vi "Sefram DAS220 - Configure and Read Channel.vi"() -> ()   [LabVIEW 2017, in "Sefram DAS220.lvlib"]
doc: "Configure an analog channel and read values."
uses:
  <instrlib>/Sefram DAS220/Sefram DAS220.lvlib
  <vilib>/Utility/error.llb/DialogType.ctl
  <instrlib>/Sefram DAS220/Public/Configure/Channels/Low-level/Set Type Voltage.vi
panel:
  in  "Channel":u16(ring) items=["A1"=0, "A2"=1, "A3"=2, "A4"=3, "A5"=4, "A6"=5, "A7"=6, "A8"=7, "A9"=8, "A10"=9, "K1"=200, "K2"=201, "K3"=202, "K4"=203, "FA1"=204, "FA2"=205, "FA3"=206, "FA4"=207]
  out "Channel":dbl(graph)
  in  "Center in Volt":dbl
  in  "Range in Volt":dbl=10.0 format="%#_13g"
  in  "stop":bool
  in  "VISA resource name":refnum<visa-resource-name>
  # "Channel Settings"
  # "Acquired Data"
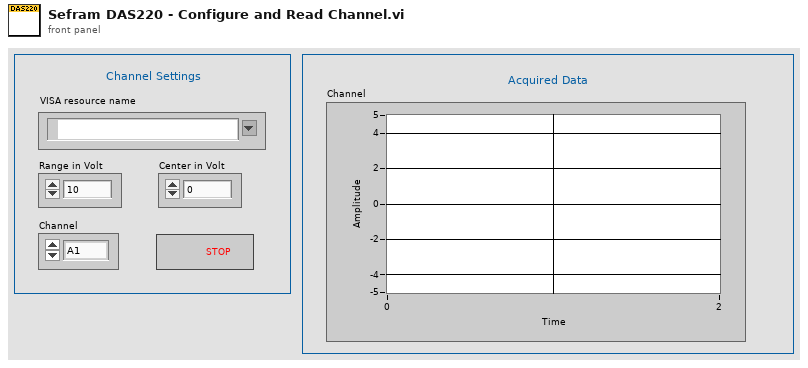
[diagram p1: front panel]
types:
  T1 = enum16{"open", "replace", "create", "open or create", "replace or create", "replace or create with confirmation"}
  T2 = typedef "DialogType.ctl" = u16
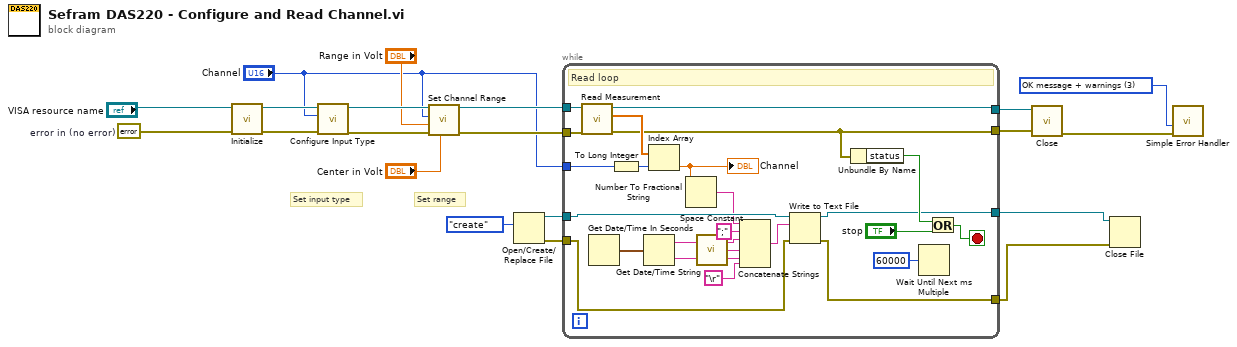
[diagram p0: block diagram]
diagram:
  w17 = errorcluster {"status"=FALSE, "code"=0, "source"=""}  # error in (no error)
  w15 = T2 3 items=["no dialog", "OK message", "continue or stop message", "OK message + warnings", "continue/stop + warnings"] ("type of dialog (OK msg:1)")
  # "Set range"
  # "Set input type"
  n1 = call <instrlib>:"Initialize.vi"("error in (no error)"=w17, "VISA resource name"="VISA resource name") -> ("error out"=w13:errorcluster, "VISA resource name out"=w14:refnum<visa-resource-name>)  [unwired: 8 in]
  n2 = call-poly <instrlib>:"Configure Input Type.vi"("error in (no error)"=w13, "Channel"="Channel", "VISA resource name"=w14) -> ("error out"=w11:errorcluster, "VISA resource name out"=w12:refnum<visa-resource-name>)  [unwired: 7 in]
  n3 = call <instrlib>:"Set Channel Range.vi"("Center (in actual channel unit)"="Center in Volt", "error in (no error)"=w11, "Channel range (in actual channel unit)"="Range in Volt", "Channel"="Channel", "VISA resource name"=w12) -> ("error out"=w10:errorcluster, "VISA resource name out"=w9:refnum<visa-resource-name>)  [unwired: 5 in]
  n4 = Open/Create/Replace File(operation (0:open)=T1."create") -> (refnum out=w6:refnum<file>, error out=w3:errorcluster)  [unwired: 5 in, 1 out]
  n5 = while {
    tunnel: [w41] -> w19
    tunnel: [w27] -> w20
    tunnel: w10 -> [w38]
    tunnel: w9 -> [w37]
    tunnel: "Channel" -> [w35]
    tunnel: w6 -> [w33]
    tunnel: [w28] -> w4
    tunnel: w3 -> [w26]
    tunnel: [w25] -> w2
    stop <- w43 stop-if-true
    # "Read loop"
    n6 = call <instrlib>:"Read Measurement.vi"("error in (no error)"=w38, "VISA resource name"=w37) -> ("error out"=w27:errorcluster, "Data"=w40:dbl[], "VISA resource name out"=w41:refnum<visa-resource-name>)  [unwired: 7 in]
    n7 = Get Date/Time In Seconds() -> (seconds since 1Jan1904=w34:timestamp)
    n8 = To Long Integer(number=w35) -> (32bit integer=w36:i32)
    n9 = Get Date/Time String(seconds (now)=w34) -> (date string=w24:string, time string=w22:string)  [unwired: 2 in]
    n10 = Index Array(array=w40, index=w36) -> (element=w32:dbl)
    "Channel" <- w32
    n11 = Number To Fractional String(number=w32) -> (F-format string=w31:string)  [unwired: 3 in]
    n12 = call <vilib>:"Space Constant.vi"() -> ("String"=w23:string)
    n13 = Concatenate Strings(w31, ";" ("string"), w24, w23, w22, "\r") -> (w29:string)
    n14 = Write to Text File(file (use dialog)=w33, text=w29, error in=w26) -> (refnum out=w28:refnum<file>, error out=w25:errorcluster)  [unwired: 1 in, 1 out]
    n15 = Unbundle By Name(w27) -> ("status"=w42:bool)
    n16 = Wait Until Next ms Multiple(millisecond multiple=u32 60000 ("milliseconds to wait")) -> ()  [unwired: 1 out]
    n17 = Or(x=w42, y="stop") -> (x .or. y?=w43:bool)
  }
  n18 = call <instrlib>:"Close.vi"("error in (no error)"=w20, "VISA resource name"=w19) -> ("error out"=w16:errorcluster)  [unwired: 9 in]
  n19 = Close File(refnum=w4, error in=w2) -> ()  [unwired: 2 out]
  n20 = call <vilib>:"Simple Error Handler.vi"("type of dialog (OK msg:1)"=w15, "error in (no error)"=w16) -> ()  [unwired: 3 in, 5 out]
